vi "Eurotherm - Setup Dialog.vi"() -> ()   [LabVIEW 2011]
uses:
  Eurotherm - Controls/Eurotherm - Setups.ctl
  Eurotherm - Controls/Eurotherm - Setup.ctl
  Eurotherm - Controls/Eurotherm - Communication.ctl
  Common/Utilities/Controls - Com Ports/Com Port - Numeric.ctl
  Eurotherm - Controls/Eurotherm - Address.ctl
  Common/Utilities/Controls - Com Ports/Com Port - Baud Rate.ctl
  Common/Utilities - System/Sensors/Sensors - Controls/Sensors - Temperature Sensor Type.ctl
  Common/Utilities - System/Sensors/Sensors - Controls/Sensors - Conversion Type.ctl
  Common/Utilities/VI Control/Control - Display State.ctl
panel:
  in  "Eurotherm Setups":T1 {"Min Set Point" format="%.3f"; "Max Set Point" format="%.3f"; "Communication"."Baud Rate" items=["300"=300, "600"=600, "1200"=1200, "2400"=2400, "4800"=4800, "9600 (default)"=9600, "19200"=19200, "38400"=38400, "57600"=57600, "76800"=76800, "115200"=115200, "230400"=230400]; "Communication"."Com Port" min=1 max=255; "Communication"."Address" min=1 max=99}
  in  "Cancel":bool
  in  "Save":bool
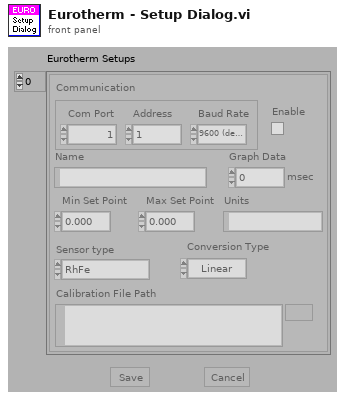
[diagram p1: front panel]
types:
  T1 = typedef "Eurotherm - Setups.ctl" = T2[]
  T2 = typedef "Eurotherm - Setup.ctl" = cluster{"Communication":T3, "Name":string, "Enable":bool, "Max Set Point":dbl, "Min Set Point":dbl, "Units":string, "Graph Data":u32, "Sensor type":T7, "Calibration File Path":path, "Conversion Type":T8}
  T3 = typedef "Eurotherm - Communication.ctl" = cluster{"Com Port":T4, "Address":T5, "Baud Rate":T6}
  T4 = typedef "Com Port - Numeric.ctl" = i32
  T5 = typedef "Eurotherm - Address.ctl" = u8
  T6 = typedef "Com Port - Baud Rate.ctl" = u32
  T7 = typedef "Sensors - Temperature Sensor Type.ctl" = enum16{"RhFe", "Pt", "K type thermocouple", "W5 type thermocouple", "No Conversion"}
  T8 = typedef "Sensors - Conversion Type.ctl" = enum16{"Linear", "Spline"}
  T9 = typedef "Control - Display State.ctl" = enum16{"Enabled", "Disabled", "Disabled and Grayed"}
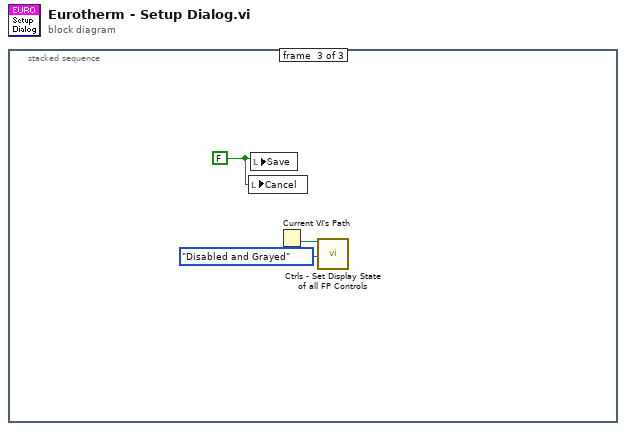
[diagram p0: block diagram]
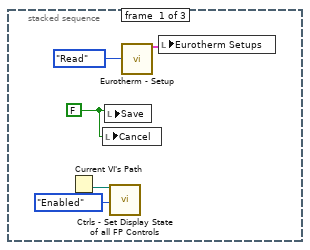
[diagram p2: hidden frame]
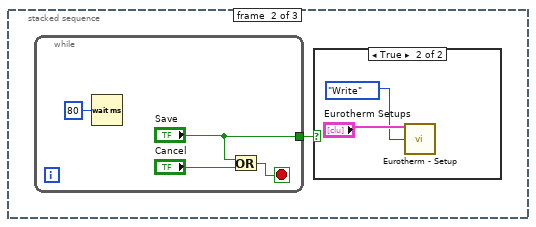
[diagram p3: hidden frame]
diagram:
  n1 = stacked-sequence {
    frame #0 {
      w5 = FALSE
      n2 = Current VI's Path() -> (path=w2:path)
      n3 = local write "Cancel"(w5) -> ()
      n4 = local write "Save"(w5) -> ()
      n5 = call "Ctrls - Set Display State of all FP Controls.vi"("VI Path"=w2, "Display State"=Control_-_Display_State."Enabled") -> ()  [unwired: 18 in]
      n6 = call "Eurotherm - Setup.vi"("Action"=enum16{"Read", "Write"}."Read") -> ("Setup Out"=w3:T1)  [unwired: 12 in, 2 out]
      n7 = local write "Eurotherm Setups"(w3) -> ()
    }
    frame #1 {
      n8 = while {
        tunnel: ["Save"] -> w6
        stop <- w11 stop-if-true
        n9 = Wait (ms)(milliseconds to wait=u32 80) -> ()  [unwired: 1 out]
        n10 = Or(x="Save", y="Cancel") -> (x .or. y?=w11:bool)
      }
      n11 = case shown="True" w6 {
        frame False {
        }
        frame True {
          n12 = call "Eurotherm - Setup.vi"("Setup In"="Eurotherm Setups", "Action"=enum16{"Read", "Write"}."Write") -> ()  [unwired: 11 in, 3 out]
        }
      }
    }
    frame #2 {
      w15 = FALSE
      n13 = local write "Cancel"(w15) -> ()
      n14 = local write "Save"(w15) -> ()
      n15 = Current VI's Path() -> (path=w14:path)
      n16 = call "Ctrls - Set Display State of all FP Controls.vi"("VI Path"=w14, "Display State"=Control_-_Display_State."Disabled and Grayed") -> ()  [unwired: 18 in]
    }
  }
